vi "Get class name.vi"(8 "error in (no error)":errorcluster caption="entrée d'erreur (pas d'erreur)", 11 "DAQmxTask en entrée":refnum<class "DAQmxTask.lvclass">) -> (0 "error out":errorcluster caption="sortie d'erreur", 2 "Class name":string, 3 "DAQmxTask en sortie":refnum<class "DAQmxTask.lvclass">)   [LabVIEW 2015, in "DAQmxTask.lvclass"]
uses:
  DAQmxTask.lvclass
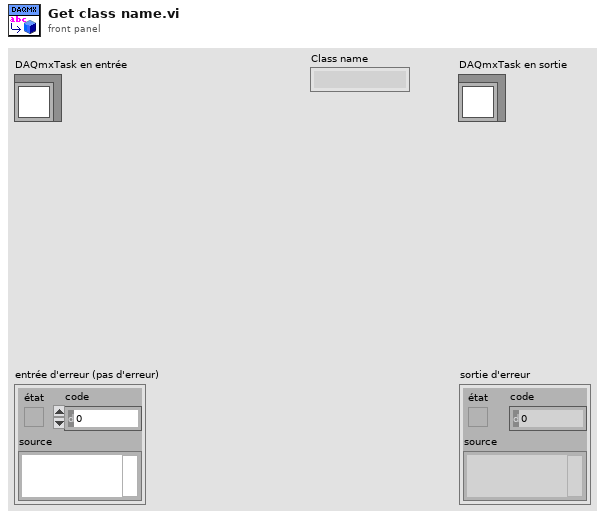
[diagram p1: front panel]
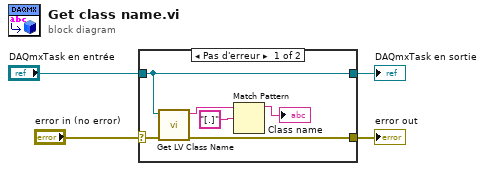
[diagram p0: block diagram]
diagram:
  n1 = case shown="Pas d'erreur" "error in (no error)" {
    selector: "error in (no error)" -> [w9 w12]
    tunnel: [w8 w12] -> w3
    tunnel: [w10 w11] -> w1
    tunnel: "DAQmxTask en entrée" -> [w10 w11]
    frame No Error {
      n2 = call <vilib>:"Get LV Class Name.vi"("error in (no error)"=w9, "object"=w10) -> ("error out"=w8:errorcluster, "class name"=w7:string)  [unwired: 8 in]
      n3 = Match Pattern(string=w7, regular expression="[.]" ("expression régulière")) -> (before substring=→"Class name":string)  [unwired: 1 in, 3 out]
    }
    frame Error {
    }
  }
  "error out" <- w3
  "DAQmxTask en sortie" <- w1
